vi "round.step.1.vi"(10 "Numeric in":u8, 11 "Array":u64[](array[numeric])) -> (3 "Numeric out":u64)   [LabVIEW 2021]
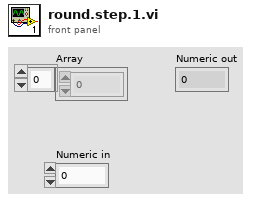
[diagram p1: front panel]
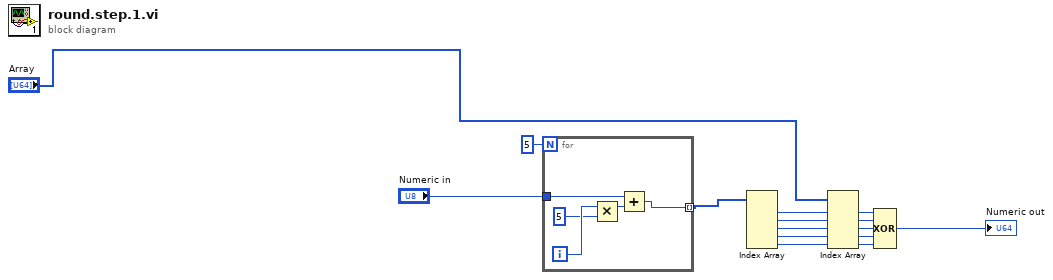
[diagram p0: block diagram]
diagram:
  n1 = for {
    N: 5 -> [_]
    tunnel: "Numeric in" -> [w19]
    tunnel: [w16] -> w3 mode=indexing
    i -> [w20]
    n2 = Multiply(x=w20, y=5) -> (x*y=w18:i32)
    n3 = Add(x=w19, y=w18) -> (x+y=w16:i32)
  }
  n4 = Index Array(array=w3) -> (element #1=w9:i32, element #2=w10:i32, element #3=w11:i32, element #4=w12:i32, element #5=w13:i32)  [unwired: 5 in]
  n5 = Index Array(array="Array", index #1=w9, index #2=w10, index #3=w11, index #4=w12, index #5=w13) -> (element #1=w4:u64, element #2=w5:u64, element #3=w6:u64, element #4=w7:u64, element #5=w8:u64)
  n6 = Compound Arithmetic op=XOR(w4, w5, w6, w7, w8) -> (→"Numeric out":u64)
